vi "fetch_generic_trigger.vi"(8 "error in (no error)":errorcluster, 11 "GenericToplevelComponent in":refnum<class "GenericToplevelComponent.lvclass">) -> (0 "error out":errorcluster, 1 "common trigger":T3, 2 "trigger":variant, 3 "GenericToplevelComponent out":refnum<class "GenericToplevelComponent.lvclass">, 4 "trigger type":T2, 5 "sender call chain":string, 6 "sender TLC type":T1=enum."ImagingMode")   [LabVIEW 2010, in "GenericToplevelComponent.lvclass"]
uses:
  GenericToplevelComponent.lvclass
  common_trigger_enum.ctl
  trigger_type_enum.ctl
  enumerations/top-level_component_type_enum.ctl
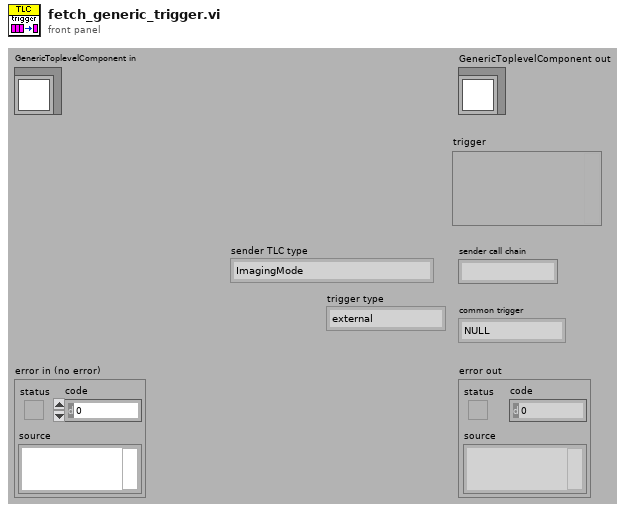
[diagram p1: front panel]
types:
  T1 = typedef "top-level_component_type_enum.ctl" = enum16{"undefined", "ImagingMode", "ScanHead", "DAQ", "ImageAssembler", "Display", "DataCollection", "Analyser", "Stimulator", "ExperimentController", "Instrument", "Stage"}
  T2 = typedef "trigger_type_enum.ctl" = enum8{"external", "internal", "common"}
  T3 = typedef "GenericToplevelComponent.lvclass/common_trigger_enum.ctl" = enum16{"NULL", "initialise", "terminate", "fetch command", "fetch data", "attach observer", "register as observer", "detach observer", "acknowledge", "start", "stop", "sweep started", "sweep finished", "experiment started", "experiment stopped"}
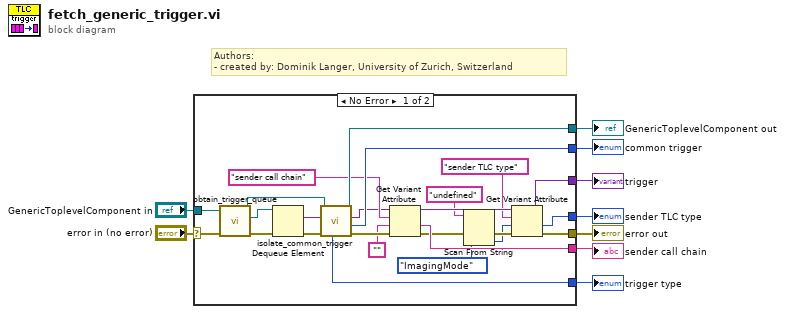
[diagram p0: block diagram]
diagram:
  # "Authors: \n- created by: Dominik Langer, University of Zurich, Switzerland"
  n1 = case shown="No Error" "error in (no error)" {
    selector: "error in (no error)" -> [w32 w36]
    tunnel: [w20 w36] -> w8
    tunnel: [w27 w35] -> w6
    tunnel: "GenericToplevelComponent in" -> [w31 w35]
    tunnel: [w17 _] -> w5
    tunnel: [w26 _] -> w4
    tunnel: [w25 _] -> w3
    tunnel: [w22 _] -> w2
    tunnel: [w15 _] -> w1
    frame No Error {
      n2 = call-dynamic "obtain_trigger_queue.vi"("error in (no error)"=w32, "GenericPlugin in"=w31) -> ("error out"=w34:errorcluster, "trigger queue"=w33:refnum<queue>, "GenericPlugin out"=w28:refnum<class "GenericToplevelComponent.lvclass">)  [unwired: 7 in]
      n3 = Dequeue Element(queue=w33, error in (no error)=w34) -> (element=w30:variant, error out=w29:errorcluster)  [unwired: 1 in, 2 out]
      n4 = call-dynamic "isolate_common_trigger.vi"("error in (no error)"=w29, "trigger variant in"=w30, "GenericToplevelComponent in"=w28) -> ("error out"=w24:errorcluster, "common trigger"=w26:T3, "trigger variant out"=w18:variant, "GenericToplevelComponent out"=w27:refnum<class "GenericToplevelComponent.lvclass">, "trigger type"=w25:T2)  [unwired: 3 in, 1 out]
      n5 = Get Variant Attribute(Variant=w18, name="sender call chain", default value (empty Variant)="", error in=w24) -> (duplicate Variant=w19:variant, value=w22:string, error out=w14:errorcluster)  [unwired: 1 out]
      n6 = Scan From String(input string="undefined" ("name"), error in=w14, default 1=top-level_component_type_enum."ImagingMode" ("top-level component type")) -> (error out=w13:errorcluster, output 1=w12:T1)  [unwired: 2 in, 2 out]
      n7 = Get Variant Attribute(Variant=w19, name="sender TLC type", default value (empty Variant)=w12, error in=w13) -> (duplicate Variant=w17:variant, value=w15:T1, error out=w20:errorcluster)  [unwired: 1 out]
    }
    frame Error {
    }
  }
  "error out" <- w8
  "GenericToplevelComponent out" <- w6
  "trigger" <- w5
  "common trigger" <- w4
  "trigger type" <- w3
  "sender call chain" <- w2
  "sender TLC type" <- w1
